vi "ARN-Protokolleinstellungen speichern.vi"(6 "Aktion":T1, 9 "Textname":string, 11 "Pfad":path) -> (1 "Textname":string, 3 "Pfad":path)   [LabVIEW 2020, in "EPA 1065.lvlib" / "ARN Test 1065-305.lvlib"]
uses:
  ARN Test 1065-305.lvlib
  Aktion FGV ARN-Protokolleinstellungen.ctl
  <vilib>/Utility/config.llb/Read Key (Path).vi
  <vilib>/Utility/config.llb/Read Key (String).vi
  <vilib>/Utility/config.llb/Write Key (Path).vi
  <vilib>/Utility/config.llb/Write Key (String).vi
  <vilib>/Utility/config.llb/NI_LVConfig.lvlib
  Allgemein/allgemeine Sub-VIs.lvlib
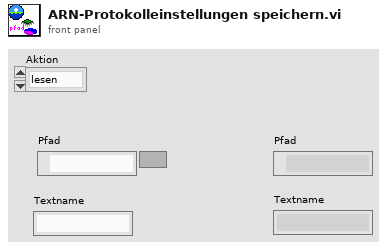
[diagram p1: front panel]
types:
  T1 = typedef "EPA 1065.lvlib/ARN Test 1065-305.lvlib/Aktion FGV ARN-Protokolleinstellungen.ctl" = enum16{"lesen", "schreiben", "laden", "speichern"}
  T2 = typedef "NI_LVConfig.lvlib/Config Data RefNum.ctl" = refnum<k1>
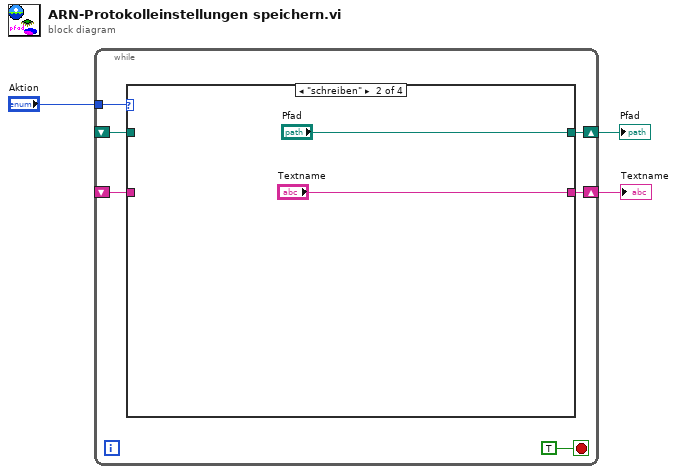
[diagram p0: block diagram]
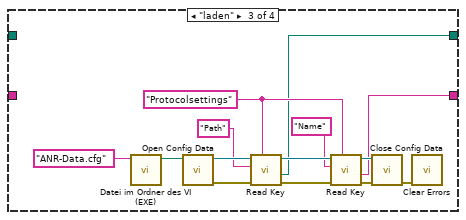
[diagram p3: hidden frame]
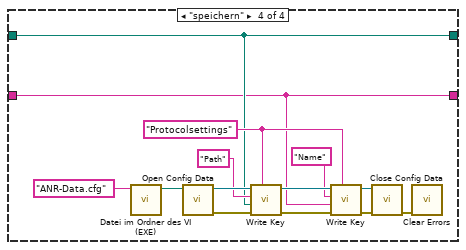
[diagram p4: hidden frame]
diagram:
  n1 = while {
    tunnel: "Aktion" -> [w8]
    shift-right: [w7] -> w2
    shift-left: _ -> [w4]
    shift-right: [w6] -> w1
    shift-left: _ -> [w5]
    stop <- TRUE stop-if-true
    n2 = case shown="\"schreiben\"" w8 {
      tunnel: [w11 "Pfad" w14 w29] -> w7
      tunnel: [w10 "Textname" w15 w28] -> w6
      tunnel: w5 -> [w10 _ _ w28]
      tunnel: w4 -> [w11 _ _ w29]
      frame "lesen", Default {
      }
      frame "schreiben" {
      }
      frame "laden" {
        w18 = "Protocolsettings" ("section")
        n3 = call "Datei im Ordner des VI (EXE).vi"("Dateiname"="ANR-Data.cfg") -> ("Dateipfad im Ordner des Haupt-VIs"=w27:path)  [unwired: 8 in, 2 out]
        n4 = call <vilib>:"Open Config Data.vi"("configuration file path"=w27) -> ("error out"=w20:errorcluster, "refnum"=w19:T2)  [unwired: 8 in, 1 out]
        n5 = call-poly <vilib>:"Read Key.vi"("section"=w18, "error in (no error)"=w20, "key"="Path", "refnum"=w19) -> ("error out"=w25:errorcluster, "value"=w14:path, "refnum out"=w24:T2)  [unwired: 4 in, 1 out]
        n6 = call-poly <vilib>:"Read Key.vi"("section"=w18, "error in (no error)"=w25, "key"="Name", "refnum"=w24) -> ("error out"=w21:errorcluster, "value"=w15:string, "refnum out"=w22:T2)  [unwired: 4 in, 1 out]
        n7 = call <vilib>:"Close Config Data.vi"("error in (no error)"=w21, "refnum"=w22) -> ("error out"=w23:errorcluster)  [unwired: 8 in, 1 out]
        n8 = call <vilib>:"Clear Errors.vi"("error in (no error)"=w23) -> ()  [unwired: 5 in, 2 out]
      }
      frame "speichern" {
        w32 = "Protocolsettings" ("section")
        n9 = call "Datei im Ordner des VI (EXE).vi"("Dateiname"="ANR-Data.cfg") -> ("Dateipfad im Ordner des Haupt-VIs"=w41:path)  [unwired: 8 in, 2 out]
        n10 = call <vilib>:"Open Config Data.vi"("configuration file path"=w41) -> ("error out"=w34:errorcluster, "refnum"=w33:T2)  [unwired: 8 in, 1 out]
        n11 = call-poly <vilib>:"Write Key.vi"("section"=w32, "error in (no error)"=w34, "value"=w29, "key"="Path", "refnum"=w33) -> ("error out"=w39:errorcluster, "refnum out"=w38:T2)  [unwired: 4 in, 1 out]
        n12 = call-poly <vilib>:"Write Key.vi"("section"=w32, "error in (no error)"=w39, "value"=w28, "key"="Name", "refnum"=w38) -> ("error out"=w35:errorcluster, "refnum out"=w36:T2)  [unwired: 4 in, 1 out]
        n13 = call <vilib>:"Close Config Data.vi"("error in (no error)"=w35, "refnum"=w36) -> ("error out"=w37:errorcluster)  [unwired: 8 in, 1 out]
        n14 = call <vilib>:"Clear Errors.vi"("error in (no error)"=w37) -> ()  [unwired: 5 in, 2 out]
      }
    }
  }
  "Pfad" <- w2
  "Textname" <- w1
